vi "LSMcontroller_v66_improvedwfhandling.vi"() -> ()   [LabVIEW 2015] (continued)
                                in-place-border: w4031 -> [w4041]
                                in-place-border: [w4038] -> w4028
                                in-place-border: [w4037] -> w4027
                                n1319 = in-place-cluster #25(w4032) -> ("aDO"=w4040:u32[])
                                n1320 = call "remove channel from active arrayv2.vi"("line array in"=w4040, "line to remove"=w4041) -> ("line array out"=w4039:u32[], "removal"=w4038:bool, "index"=w4037:i32)
                                n1321 = in-place-cluster #25("aDO"=w4039) -> (w4029:T10)
                                }
                                n1322 = call "2pparameters.vi"("Params in"=w4029, "command"="set") -> ()  [unwired: 1 out]
                                }
                                frame True {
                                }
                                }
                                }
                                frame True {
                                n1323 = call "configuration.vi"("command"="get") -> ("config out"=w4048:T11)  [unwired: 2 in, 1 out]
                                n1324 = call "2pparameters.vi"("command"="get") -> ("params out"=w4052:T10)  [unwired: 1 in]
                                n1325 = Unbundle By Name(w4048) -> ("2P shutter"=w4047:i32)
                                n1326 = in-place {
                                in-place-border: w4047 -> [w4058]
                                in-place-border: [w4055] -> w4046
                                in-place-border: [w4054] -> w4044
                                n1327 = in-place-cluster #26(w4052) -> ("aDO"=w4057:u32[])
                                n1328 = call "add channel to active arrayv2.vi"("line array in"=w4057, "line to add"=w4058) -> ("line array out"=w4056:u32[], "addition"=w4055:bool, "index"=w4054:i32)
                                n1329 = in-place-cluster #26("aDO"=w4056) -> (w4050:T10)
                                }
                                n1330 = call "2pparameters.vi"("Params in"=w4050, "command"="set") -> ()  [unwired: 1 out]
                                }
                                }
                                }
                                frame #3 {
                                n1331 = local read "Measurement"() -> (w4062:T4)
                                n1332 = To Unsigned Long Integer(number=w4062) -> (unsigned 32bit integer=w4063:u32)
                                n1333 = case shown="5..7" w4063 {
                                tunnel: [FALSE ("addition") w4081] -> w4061
                                tunnel: [w4066 FALSE ("removal")] -> w4060
                                tunnel: [w4064 w4079] -> w4059
                                frame 0..4, Default {
                                n1334 = call "configuration.vi"("command"="get") -> ("config out"=w4072:T11)  [unwired: 2 in, 1 out]
                                n1335 = Unbundle By Name(w4072) -> ("LT timestamp"=w4069:u32)
                                n1336 = call "2pparameters.vi"("command"="get") -> ("params out"=w4070:T10)  [unwired: 1 in]
                                n1337 = in-place {
                                in-place-border: w4069 -> [w4078]
                                in-place-border: [w4075] -> w4066
                                in-place-border: [w4074] -> w4064
                                n1338 = in-place-cluster #27(w4070) -> ("aDO"=w4077:u32[])
                                n1339 = call "remove channel from active arrayv2.vi"("line array in"=w4077, "line to remove"=w4078) -> ("line array out"=w4076:u32[], "removal"=w4075:bool, "index"=w4074:i32)
                                n1340 = in-place-cluster #27("aDO"=w4076) -> (w4067:T10)
                                }
                                n1341 = call "2pparameters.vi"("Params in"=w4067, "command"="set") -> ()  [unwired: 1 out]
                                }
                                frame 5..7 {
                                n1342 = call "configuration.vi"("command"="get") -> ("config out"=w4087:T11)  [unwired: 2 in, 1 out]
                                n1343 = Unbundle By Name(w4087) -> ("LT timestamp"=w4084:u32)
                                n1344 = call "2pparameters.vi"("command"="get") -> ("params out"=w4085:T10)  [unwired: 1 in]
                                n1345 = in-place {
                                in-place-border: w4084 -> [w4093]
                                in-place-border: [w4090] -> w4081
                                in-place-border: [w4089] -> w4079
                                n1346 = in-place-cluster #28(w4085) -> ("aDO"=w4092:u32[])
                                n1347 = call "add channel to active arrayv2.vi"("line array in"=w4092, "line to add"=w4093) -> ("line array out"=w4091:u32[], "addition"=w4090:bool, "index"=w4089:i32)
                                n1348 = in-place-cluster #28("aDO"=w4091) -> (w4082:T10)
                                }
                                n1349 = call "2pparameters.vi"("Params in"=w4082, "command"="set") -> ()  [unwired: 1 out]
                                }
                                }
                                }
                                }
                                }
                                frame #1 {
                                n1350 = Or(x=w4100, y=w4101) -> (x .or. y?=w4099:bool)
                                n1351 = case shown="True" w4099 {
                                frame False {
                                }
                                frame True {
                                # "update GUI"
                                n1352 = call "Used AO lines.vi"() -> ("used AO names"=w4105:string[], "used AO lines"=w4107:tag[])  [unwired: 2 in]
                                n1353 = control-ref of="Analog Lines Plot"() -> (w4106:refnum<vi>)
                                n1354 = local write "Analog Used Lines"(w4107) -> ()
                                n1355 = local write "Analog Used Names"(w4105) -> ()
                                n1356 = call "prepAOWaveplot.vi"("WaveformGraph in"=w4106, "Analog Used Names"=w4105) -> ()  [unwired: 1 in]
                                }
                                }
                                n1357 = Compound Arithmetic op=OR(w4097, w4096, w4095, w4094) -> (w4098:bool)
                                n1358 = case shown="True" w4098 {
                                frame False {
                                }
                                frame True {
                                n1359 = control-ref of="Digital Lines Plot"() -> (w4102:refnum<vi>)
                                n1360 = call "Used DO lines.vi"() -> ("used DO names"=w4103:string[], "used DO lines"=w4104:tag[])  [unwired: 2 in]
                                n1361 = local write "Digital Used Lines"(w4104) -> ()
                                n1362 = local write "Digital Used Names"(w4103) -> ()
                                n1363 = call "prepDOWaveplot.vi"("DigitalGraph in"=w4102, "used DO names"=w4103) -> ()  [unwired: 1 in]
                                }
                                }
                                }
                                frame #2 {
                                n1364 = case shown="False" w4111 {
                                tunnel: [w4114 w4140] -> w4110
                                tunnel: [w4113 w4138] -> w4109
                                tunnel: [w4112 _] -> w4108
                                frame False {
                                n1365 = stacked-sequence {
                                seq-local: [w4116 _] -> [_ w4131]
                                tunnel: [w4116 _] -> w4114
                                tunnel: [w4119 _] -> w4113
                                tunnel: [w4115 _] -> w4112
                                frame #0 {
                                n1366 = call "configuration.vi"("command"="get") -> ("config out"=w4127:T11)  [unwired: 2 in, 1 out]
                                n1367 = call "waveformparamsv2.vi"("command"="get") -> ("Params out"=w4121:T14)  [unwired: 4 in, 2 out]
                                n1368 = Unbundle By Name(w4127) -> ("Voltage to Xgalvo"=w4128:i32)
                                n1369 = call "2pparameters.vi"("command"="get") -> ("params out"=w4124:T10)  [unwired: 1 in]
                                n1370 = Unbundle By Name(w4121) -> ("AO parameters"=w4120:T15)
                                n1371 = Unbundle By Name(w4124) -> ("aAO"=w4125:u32[])
                                n1372 = call "waveformsAObuffer.vi"("command"="get") -> ("AO wf out"=w4117:waveform(dbl)[])  [unwired: 1 in]
                                n1373 = Search 1D Array(1D array=w4125, element=w4128) -> (index of element=w4116:i32)  [unwired: 1 in]
                                n1374 = Index Array(array=w4117, index=w4116) -> (element=w4115:waveform(dbl))
                                n1375 = Index Array(array=w4120, index=w4116) -> (element=w4119:T16)
                                }
                                frame #1 {
                                w4132 = 0.0 ("Step size (V)")
                                n1376 = local read "Meastab"() -> (w4130:enum32{"X-Y Image", "Linescan", "Timetrace"})
                                n1377 = case shown="\"X-Y Image\", Default" w4130 {
                                tunnel: [w4134 w4135] -> w4129
                                frame "X-Y Image", Default {
                                n1378 = local read "Sampling rate"() -> (w4134:dbl)
                                }
                                frame "Timetrace" {
                                n1379 = local read "srateAODOtt"() -> (w4135:dbl)
                                }
                                }
                                n1380 = call "replace AO XYwfparam.vi"("Baseline (V)"=w4132, "Start amplitude (V)"=w4132, "Cycles"=w4132, "Repeats"=w4132, "index of AO wave"=w4131, "Step size (V)"=w4132, "DC (%)"=w4132, "Sampling frequency (Hz)"=w4129, "Period (ms)"=w4132, "Cycle length (s)"=w4132, "Pulses"=w4132, "padding value"=w4132, "Matlab wave name"=path "xwave") -> ()  [unwired: 3 in]
                                }
                                }
                                }
                                frame True {
                                w4139 = 0.0 ("Repeats")
                                n1381 = local read "Meastab"() -> (w4137:enum32{"X-Y Image", "Linescan", "Timetrace"})
                                n1382 = case shown="\"X-Y Image\", Default" w4137 {
                                tunnel: [w4156 w4157] -> w4136
                                frame "X-Y Image", Default {
                                n1383 = local read "Sampling rate"() -> (w4156:dbl)
                                }
                                frame "Timetrace" {
                                n1384 = local read "srateAODOtt"() -> (w4157:dbl)
                                }
                                }
                                n1385 = call "2pparameters.vi"("command"="get") -> ("params out"=w4142:T10)  [unwired: 1 in]
                                n1386 = call "configuration.vi"("command"="get") -> ("config out"=w4145:T11)  [unwired: 2 in, 1 out]
                                n1387 = call "waveformparamsv2.vi"("command"="get") -> ("Params out"=w4153:T14)  [unwired: 4 in, 2 out]
                                n1388 = Unbundle By Name(w4145) -> ("Voltage to Xgalvo"=w4146:i32)
                                n1389 = Unbundle By Name(w4153) -> ("AO parameters"=w4150:T15)
                                n1390 = Unbundle By Name(w4142) -> ("aAO"=w4143:u32[])
                                n1391 = Search 1D Array(1D array=w4143, element=w4146) -> (index of element=w4140:i32)  [unwired: 1 in]
                                n1392 = Index Array(array=w4150, index=0) -> (element=w4151:T16)
                                n1393 = Bundle By Name(cluster=w4151, "AOtab"=-1.0 ("Repeats"), "Repeats"=w4139, "Cycles"=w4139, "Start amplitude (V)"=w4139, "Baseline (V)"=w4139, "Step size (V)"=w4139, "DC (%)"=w4139, "Sampling frequency (Hz)"=w4136, "Period (ms)"=w4139, "Offset (V)"=w4139, "Amplitude (V)"=w4139, "Frequency"=w4139, "Tri Repeats"=w4139, "phase shift (ms)"=w4139, "Pulses"=w4139, "Matlab wave file"=path "xwave", "padding value"=w4139) -> (w4138:T16)
                                n1394 = Build Array(w4138) -> (w4148:T15)
                                n1395 = call "waveformparamsv2.vi"("command"="add AO", "add AO"=w4148) -> ()  [unwired: 3 in, 3 out]
                                }
                                }
                                }
                                frame #3 {
                                n1396 = case shown="False" w4161 {
                                tunnel: [w4164 w4190] -> w4160
                                tunnel: [w4163 w4188] -> w4159
                                tunnel: [w4162 _] -> w4158
                                frame False {
                                n1397 = stacked-sequence {
                                seq-local: [w4166 _] -> [_ w4181]
                                tunnel: [w4166 _] -> w4164
                                tunnel: [w4169 _] -> w4163
                                tunnel: [w4165 _] -> w4162
                                frame #0 {
                                n1398 = call "configuration.vi"("command"="get") -> ("config out"=w4177:T11)  [unwired: 2 in, 1 out]
                                n1399 = call "waveformparamsv2.vi"("command"="get") -> ("Params out"=w4171:T14)  [unwired: 4 in, 2 out]
                                n1400 = Unbundle By Name(w4177) -> ("Voltage to Ygalvo"=w4178:i32)
                                n1401 = call "2pparameters.vi"("command"="get") -> ("params out"=w4174:T10)  [unwired: 1 in]
                                n1402 = Unbundle By Name(w4171) -> ("AO parameters"=w4170:T15)
                                n1403 = Unbundle By Name(w4174) -> ("aAO"=w4175:u32[])
                                n1404 = call "waveformsAObuffer.vi"("command"="get") -> ("AO wf out"=w4167:waveform(dbl)[])  [unwired: 1 in]
                                n1405 = Search 1D Array(1D array=w4175, element=w4178) -> (index of element=w4166:i32)  [unwired: 1 in]
                                n1406 = Index Array(array=w4167, index=w4166) -> (element=w4165:waveform(dbl))
                                n1407 = Index Array(array=w4170, index=w4166) -> (element=w4169:T16)
                                }
                                frame #1 {
                                w4182 = 0.0 ("Step size (V)")
                                n1408 = local read "Meastab"() -> (w4180:enum32{"X-Y Image", "Linescan", "Timetrace"})
                                n1409 = case shown="\"X-Y Image\", Default" w4180 {
                                tunnel: [w4184 w4185] -> w4179
                                frame "X-Y Image", Default {
                                n1410 = local read "Sampling rate"() -> (w4184:dbl)
                                }
                                frame "Timetrace" {
                                n1411 = local read "srateAODOtt"() -> (w4185:dbl)
                                }
                                }
                                n1412 = call "replace AO XYwfparam.vi"("Baseline (V)"=w4182, "Start amplitude (V)"=w4182, "Cycles"=w4182, "Repeats"=w4182, "index of AO wave"=w4181, "Step size (V)"=w4182, "DC (%)"=w4182, "Sampling frequency (Hz)"=w4179, "Period (ms)"=w4182, "Cycle length (s)"=w4182, "Pulses"=w4182, "padding value"=w4182, "Matlab wave name"=path "ywave") -> ()  [unwired: 3 in]
                                }
                                }
                                }
                                frame True {
                                w4189 = 0.0 ("Repeats")
                                n1413 = local read "Meastab"() -> (w4187:enum32{"X-Y Image", "Linescan", "Timetrace"})
                                n1414 = case shown="\"X-Y Image\", Default" w4187 {
                                tunnel: [w4206 w4207] -> w4186
                                frame "X-Y Image", Default {
                                n1415 = local read "Sampling rate"() -> (w4206:dbl)
                                }
                                frame "Timetrace" {
                                n1416 = local read "srateAODOtt"() -> (w4207:dbl)
                                }
                                }
                                n1417 = call "2pparameters.vi"("command"="get") -> ("params out"=w4192:T10)  [unwired: 1 in]
                                n1418 = call "configuration.vi"("command"="get") -> ("config out"=w4195:T11)  [unwired: 2 in, 1 out]
                                n1419 = call "waveformparamsv2.vi"("command"="get") -> ("Params out"=w4204:T14)  [unwired: 4 in, 2 out]
                                n1420 = Unbundle By Name(w4195) -> ("Voltage to Ygalvo"=w4196:i32)
                                n1421 = Unbundle By Name(w4204) -> ("AO parameters"=w4201:T15)
                                n1422 = Unbundle By Name(w4192) -> ("aAO"=w4193:u32[])
                                n1423 = Search 1D Array(1D array=w4193, element=w4196) -> (index of element=w4190:i32)  [unwired: 1 in]
                                n1424 = Index Array(array=w4201, index=0) -> (element=w4202:T16)
                                n1425 = Bundle By Name(cluster=w4202, "AOtab"=-1.0 ("Repeats"), "Repeats"=w4189, "Cycles"=w4189, "Start amplitude (V)"=w4189, "Baseline (V)"=w4189, "Step size (V)"=w4189, "DC (%)"=w4189, "Sampling frequency (Hz)"=w4186, "Period (ms)"=w4189, "Offset (V)"=w4189, "Amplitude (V)"=w4189, "Frequency"=w4189, "Tri Repeats"=w4189, "phase shift (ms)"=w4189, "Pulses"=w4189, "Matlab wave file"=path "ywave", "padding value"=w4189) -> (w4188:T16)
                                n1426 = Build Array(w4188) -> (w4199:T15)
                                n1427 = call "waveformparamsv2.vi"("command"="add AO", "add AO"=w4199) -> ()  [unwired: 3 in, 3 out]
                                }
                                }
                                }
                                frame #4 {
                                n1428 = call "2pparameters.vi"("command"="get") -> ("params out"=w4213:T10)  [unwired: 1 in]
                                n1429 = Unbundle By Name(w4213) -> ("wavdet"=w4212:bool, "Pel"=w4209:sgl, "refwfsize"=w4208:dbl, "srateAODO"=w4211:sgl)
                                n1430 = case shown="True" w4212 {
                                tunnel: [w4217 w4227] -> w4215
                                tunnel: w4211 -> [w4218 w4229]
                                tunnel: w4209 -> [_ w4225]
                                tunnel: w4208 -> [_ w4224]
                                frame False {
                                n1431 = call "X-array-databuffer.vi"("command"=enum16{"get", "set", "clear", "append"}."get") -> ("array out"=w4221:dbl[])  [unwired: 3 in, 1 out]
                                n1432 = Reciprocal(x=w4218) -> (1/x=w4219:sgl)
                                n1433 = Bundle By Name("Y"=w4221, "dt"=w4219) -> (w4217:waveform(dbl))  [unwired: 1 in]
                                }
                                frame True {
                                n1434 = To Double Precision Float(number=w4225) -> (double precision float=w4226:dbl)
                                n1435 = Divide(x=w4224, y=w4226) -> (x/y=w4223:dbl)
                                n1436 = Round Toward +Infinity(x=w4223) -> (ceil(x): smallest int >= x=w4222:dbl)
                                n1437 = call "X-array-databuffer.vi"("command"=enum16{"get", "set", "clear", "append"}."get") -> ("array out"=w4231:dbl[])  [unwired: 3 in, 1 out]
                                n1438 = Reciprocal(x=w4229) -> (1/x=w4230:sgl)
                                n1439 = for {
                                N: w4222 -> [_]
                                tunnel: w4231 -> [w4233]
                                tunnel: [w4233] -> w4228 mode=concatenating
                                }
                                n1440 = Bundle By Name("Y"=w4228, "dt"=w4230) -> (w4227:waveform(dbl))  [unwired: 1 in]
                                }
                                }
                                n1441 = case shown="True" w4216 {
                                tunnel: w4215 -> [w4235 w4241]
                                tunnel: w4210 -> [w4236 _]
                                frame False {
                                n1442 = call "waveformsAObuffer.vi"("command"="get") -> ("AO wf out"=w4239:waveform(dbl)[])  [unwired: 1 in]
                                n1443 = property on="refwf" class="Ring (strict)" props=["RingText", "Text"]() -> ()  [unwired: 2 in, 3 out]
                                n1444 = Replace Array Subset(array=w4239, new element=w4235, index=w4236) -> (w4234:waveform(dbl)[])
                                n1445 = call "waveformsAObuffer.vi"("AO wf in"=w4234, "command"="set") -> ()  [unwired: 1 out]
                                }
                                frame True {
                                n1446 = call "waveformsAObuffer.vi"("command"="get") -> ("AO wf out"=w4243:waveform(dbl)[])  [unwired: 1 in]
                                n1447 = Build Array (concatenate)(w4243, w4241) -> (w4240:waveform(dbl)[])
                                n1448 = call "waveformsAObuffer.vi"("AO wf in"=w4240, "command"="set") -> ()  [unwired: 1 out]
                                }
                                }
                                }
                                frame #5 {
                                n1449 = call "2pparameters.vi"("command"="get") -> ("params out"=w4255:T10)  [unwired: 1 in]
                                n1450 = Unbundle By Name(w4255) -> ("wavdet"=w4254:bool, "Pel"=w4252:sgl, "refwfsize"=w4253:dbl, "srateAODO"=w4248:sgl)
                                n1451 = To Double Precision Float(number=w4252) -> (double precision float=w4251:dbl)
                                n1452 = Divide(x=w4253, y=w4251) -> (x/y=w4250:dbl)
                                n1453 = Round Toward +Infinity(x=w4250) -> (ceil(x): smallest int >= x=w4249:dbl)
                                n1454 = case shown="True" w4254 {
                                tunnel: [w4259 w4265] -> w4245
                                tunnel: w4249 -> [_ w4262]
                                tunnel: w4248 -> [w4260 w4267]
                                frame False {
                                n1455 = call "Y-array-databuffer.vi"("command"=enum16{"get", "set", "clear", "append"}."get") -> ("array out"=w4257:dbl[])  [unwired: 3 in, 1 out]
                                n1456 = Reciprocal(x=w4260) -> (1/x=w4261:sgl)
                                n1457 = Bundle By Name("Y"=w4257, "dt"=w4261) -> (w4259:waveform(dbl))  [unwired: 1 in]
                                }
                                frame True {
                                n1458 = call "Y-array-databuffer.vi"("command"=enum16{"get", "set", "clear", "append"}."get") -> ("array out"=w4263:dbl[])  [unwired: 3 in, 1 out]
                                n1459 = Reciprocal(x=w4267) -> (1/x=w4268:sgl)
                                n1460 = for {
                                N: w4262 -> [_]
                                tunnel: w4263 -> [w4269]
                                tunnel: [w4269] -> w4266 mode=concatenating
                                }
                                n1461 = Bundle By Name("Y"=w4266, "dt"=w4268) -> (w4265:waveform(dbl))  [unwired: 1 in]
                                }
                                }
                                n1462 = case shown="False" w4247 {
                                tunnel: w4245 -> [w4272 w4277]
                                tunnel: w4246 -> [w4273 _]
                                frame False {
                                n1463 = call "waveformsAObuffer.vi"("command"="get") -> ("AO wf out"=w4275:waveform(dbl)[])  [unwired: 1 in]
                                n1464 = Replace Array Subset(array=w4275, new element=w4272, index=w4273) -> (w4270:waveform(dbl)[])
                                n1465 = call "waveformsAObuffer.vi"("AO wf in"=w4270, "command"="set") -> ()  [unwired: 1 out]
                                }
                                frame True {
                                n1466 = call "waveformsAObuffer.vi"("command"="get") -> ("AO wf out"=w4279:waveform(dbl)[])  [unwired: 1 in]
                                n1467 = Build Array (concatenate)(w4279, w4277) -> (w4276:waveform(dbl)[])
                                n1468 = call "waveformsAObuffer.vi"("AO wf in"=w4276, "command"="set") -> ()  [unwired: 1 out]
                                }
                                }
                                }
                                frame #6 {
                                n1469 = Build Array(w4284, w4283) -> (w4287:bool[])
                                n1470 = Boolean Array To Number(Boolean array=w4287) -> (number=w4286:u32)
                                n1471 = case shown="2" w4286 {
                                tunnel: w4285 -> [_ _ _ _]
                                tunnel: w4282 -> [_ w4310 _ w4323]
                                tunnel: [_ w4309 _ w4320] -> w4281
                                frame 1 {
                                w4297 = 0.0 ("DOtab")
                                n1472 = call "2pparameters.vi"("command"="get") -> ("params out"=w4294:T10)  [unwired: 1 in]
                                n1473 = call "waveformparamsv2.vi"("command"="get") -> ("Params out"=w4305:T14)  [unwired: 4 in, 2 out]
                                n1474 = Unbundle By Name(w4305) -> ("DO parameters"=w4303:T17)
                                n1475 = Unbundle By Name(w4294) -> ("srate"=w4290:sgl, "Pel"=w4293:sgl)
                                n1476 = To Double Precision Float(number=w4290) -> (double precision float=w4288:dbl)
                                n1477 = To Double Precision Float(number=w4290) -> (double precision float=w4289:dbl)
                                n1478 = To Double Precision Float(number=w4293) -> (double precision float=w4292:dbl)
                                n1479 = Divide(x=w4289, y=w4292) -> (x/y=w4291:dbl)
                                n1480 = Index Array(array=w4303, index=0) -> (element=w4302:T18)
                                n1481 = Bundle By Name(cluster=w4302, "Digital DC (%)"=100.0, "Digital phase"=w4297, "Digital Freq (Hz)"=w4291, "Sampling frequency (Hz)"=w4288, "Digital time offset (s)"=w4297, "padding value"=0.0, "matlab wave file"=path "2Pshutter", "DOtab"=0.0) -> (w4300:T18)
                                n1482 = Build Array(w4300) -> (w4299:T17)
                                n1483 = call "waveformparamsv2.vi"("command"="add DO", "add DO"=w4299) -> ()  [unwired: 3 in, 3 out]
                                }
                                frame 2 {
                                n1484 = call "waveformparamsv2.vi"("command"="get") -> ("Params out"=w4312:T14)  [unwired: 4 in, 2 out]
                                n1485 = in-place {
                                in-place-border: w4310 -> [w4316]
                                in-place-border: [w4315] -> w4309
                                n1486 = in-place-cluster #29(w4312) -> ("DO parameters"=w4318:T17)
                                n1487 = Delete From Array(array=w4318, length=1, index=w4316) -> (deleted portion=w4315:T17, array with subset deleted=w4317:T17)
                                n1488 = in-place-cluster #29("DO parameters"=w4317) -> (w4311:T14)
                                }
                                n1489 = call "waveformparamsv2.vi"("command"="set", "Params in"=w4311) -> ()  [unwired: 3 in, 3 out]
                                }
                                frame 3, Default {
                                }
                                frame 0 {
                                n1490 = call "2pparameters.vi"("command"="get") -> ("params out"=w4325:T10)  [unwired: 1 in]
                                n1491 = Unbundle By Name(w4325) -> ("wavdet"=w4322:bool, "autoshutter"=w4324:bool)
                                n1492 = case shown="True" w4324 {
                                tunnel: w4323 -> [_ w4329]
                                tunnel: w4322 -> [_ w4328]
                                tunnel: [_ w4327] -> w4321
                                frame False {
                                }
                                frame True {
                                n1493 = case shown="False" w4328 {
                                tunnel: w4329 -> [w4331 _]
                                tunnel: [w4330 _] -> w4327
                                frame False {
                                n1494 = stacked-sequence {
                                tunnel: w4331 -> [w4333 w4347]
                                tunnel: [w4332 _] -> w4330
                                frame #0 {
                                n1495 = call "waveformparamsv2.vi"("command"="get") -> ("Params out"=w4335:T14)  [unwired: 4 in, 2 out]
                                n1496 = Unbundle By Name(w4335) -> ("DO parameters"=w4334:T17)
                                n1497 = Index Array(array=w4334, index=w4333) -> (element=w4332:T18)
                                }
                                frame #1 {
                                w4346 = 0.0 ("padding value")
                                n1498 = call "2pparameters.vi"("command"="get") -> ("params out"=w4344:T10)  [unwired: 1 in]
                                n1499 = Unbundle By Name(w4344) -> ("srate"=w4341:sgl, "Pel"=w4343:sgl)
                                n1500 = To Double Precision Float(number=w4341) -> (double precision float=w4339:dbl)
                                n1501 = To Double Precision Float(number=w4341) -> (double precision float=w4340:dbl)
                                n1502 = To Double Precision Float(number=w4343) -> (double precision float=w4342:dbl)
                                n1503 = Divide(x=w4340, y=w4342) -> (x/y=w4338:dbl)
                                n1504 = call "replace DO wf param.vi"("Digital Freq (Hz)"=w4338, "Digital DC (%)"=100.0, "Digital phase"=w4346, "Sampling frequency (Hz)"=w4339, "Digital time offset (s)"=w4346, "index of DO wave"=w4347, "padding value"=w4346, "matlab wave file"=path "2Pshutter" ("matlab wave number")) -> ()  [unwired: 3 in]
                                }
                                }
                                }
                                frame True {
                                }
                                }
                                }
                                }
                                n1505 = Build Array(w4321) -> (w4320:T17)
                                }
                                }
                                }
                                frame #7 {
                                n1506 = Build Array(w4352, w4351) -> (w4354:bool[])
                                n1507 = Boolean Array To Number(Boolean array=w4354) -> (number=w4353:u32)
                                n1508 = case shown="0" w4353 {
                                tunnel: w4350 -> [_ w4396 _ w4403]
                                tunnel: [_ w4395 _ w4401] -> w4349
                                frame 1 {
                                n1509 = call "2pparameters.vi"("command"="get") -> ("params out"=w4361:T10)  [unwired: 1 in]
                                n1510 = Unbundle By Name(w4361) -> ("wavdet"=w4362:bool, "Pel"=w4364:sgl, "refwfsize"=w4365:dbl, "srateAODO"=w4363:sgl)
                                n1511 = call "waveformsDObuffer.vi"("command"="get") -> ("DO wf out"=w4357:digitalwaveform[])  [unwired: 1 in]
                                n1512 = case shown="False" w4362 {
                                tunnel: [w4370 w4380] -> w4359
                                tunnel: w4363 -> [w4375 w4391]
                                tunnel: w4364 -> [w4369 w4384]
                                tunnel: w4365 -> [_ w4388]
                                frame False {
                                w4373 = u16 0 items=["unsigned binary", "offset binary", "2's complement"] ("data format (offset binary)")
                                n1513 = Initialize Array(sgl 1.0, w4369) -> (w4366:sgl[])
                                n1514 = Reciprocal(x=w4375) -> (1/x=w4376:sgl)
                                n1515 = Bundle By Name("Y"=w4366, "dt"=w4376) -> (w4371:waveform(sgl))  [unwired: 1 in]
                                n1516 = call-poly <vilib>:"Analog to Digital.vi"("data format (offset binary)"=w4373, "compress digital (T)"=TRUE, "full-scale range (pk-pk)"=1.0, "resolution (16 bit)"=1, "analog waveform"=w4371) -> ("digital waveform"=w4370:digitalwaveform)  [unwired: 3 in, 3 out]
                                }
                                frame True {
                                w4383 = u16 0 items=["unsigned binary", "offset binary", "2's complement"] ("data format (offset binary)")
                                n1517 = To Double Precision Float(number=w4384) -> (double precision float=w4389:dbl)
                                n1518 = Initialize Array(sgl 1.0, w4384) -> (w4377:sgl[])
                                n1519 = Divide(x=w4388, y=w4389) -> (x/y=w4386:dbl)
                                n1520 = Round Toward +Infinity(x=w4386) -> (ceil(x): smallest int >= x=w4387:dbl)
                                n1521 = for {
                                N: w4387 -> [_]
                                tunnel: w4377 -> [w4393]
                                tunnel: [w4393] -> w4390 mode=concatenating
                                }
                                n1522 = Reciprocal(x=w4391) -> (1/x=w4392:sgl)
                                n1523 = Bundle By Name("Y"=w4390, "dt"=w4392) -> (w4381:waveform(sgl))  [unwired: 1 in]
                                n1524 = call-poly <vilib>:"Analog to Digital.vi"("data format (offset binary)"=w4383, "compress digital (T)"=TRUE, "full-scale range (pk-pk)"=1.0, "resolution (16 bit)"=1, "analog waveform"=w4381) -> ("digital waveform"=w4380:digitalwaveform)  [unwired: 3 in, 3 out]
                                }
                                }
                                n1525 = Build Array (concatenate)(w4357, w4359) -> (w4355:digitalwaveform[])
                                n1526 = call "waveformsDObuffer.vi"("DO wf in"=w4355, "command"="set") -> ()  [unwired: 1 out]
                                }
                                frame 2 {
                                n1527 = call "waveformsDObuffer.vi"("command"="get") -> ("DO wf out"=w4398:digitalwaveform[])  [unwired: 1 in]
                                n1528 = Delete From Array(array=w4398, length=1, index=w4396) -> (deleted portion=w4395:digitalwaveform[], array with subset deleted=w4394:digitalwaveform[])
                                n1529 = call "waveformsDObuffer.vi"("DO wf in"=w4394, "command"="set") -> ()  [unwired: 1 out]
                                }
                                frame 3, Default {
                                }
                                frame 0 {
                                n1530 = call "2pparameters.vi"("command"="get") -> ("params out"=w4405:T10)  [unwired: 1 in]
                                n1531 = Unbundle By Name(w4405) -> ("autoshutter"=w4404:bool, "wavdet"=w4402:bool)
                                n1532 = case shown="True" w4404 {
                                tunnel: w4403 -> [_ w4409]
                                tunnel: w4402 -> [_ w4408]
                                tunnel: [_ w4407] -> w4401
                                frame False {
                                }
                                frame True {
                                n1533 = case shown="False" w4408 {
                                tunnel: w4409 -> [w4413 _]
                                tunnel: [w4411 _] -> w4407
                                frame False {
                                w4420 = u16 0 items=["unsigned binary", "offset binary", "2's complement"] ("data format (offset binary)")
                                n1534 = call "2pparameters.vi"("command"="get") -> ("params out"=w4427:T10)  [unwired: 1 in]
                                n1535 = call "waveformsDObuffer.vi"("command"="get") -> ("DO wf out"=w4414:digitalwaveform[])  [unwired: 1 in]
                                n1536 = Unbundle By Name(w4427) -> ("Pel"=w4429:sgl, "srate"=w4428:sgl)
                                n1537 = Index Array(array=w4414, index=w4413) -> (element=w4412:digitalwaveform)
                                n1538 = Build Array(w4412) -> (w4411:digitalwaveform[])
                                n1539 = Initialize Array(sgl 1.0, w4429) -> (w4415:sgl[])
                                n1540 = Reciprocal(x=w4428) -> (1/x=w4422:sgl)
                                n1541 = Bundle By Name("Y"=w4415, "dt"=w4422) -> (w4418:waveform(sgl))  [unwired: 1 in]
                                n1542 = call-poly <vilib>:"Analog to Digital.vi"("data format (offset binary)"=w4420, "compress digital (T)"=TRUE, "full-scale range (pk-pk)"=1.0, "resolution (16 bit)"=1, "analog waveform"=w4418) -> ("digital waveform"=w4425:digitalwaveform)  [unwired: 3 in, 3 out]
                                n1543 = Replace Array Subset(array=w4414, new element=w4425, index=w4413) -> (w4410:digitalwaveform[])
                                n1544 = call "waveformsDObuffer.vi"("DO wf in"=w4410, "command"="set") -> ()  [unwired: 1 out]
                                }
                                frame True {
                                }
                                }
                                }
                                }
                                }
                                }
                                }
                                frame #8 {
                                n1545 = Build Array(w4433, w4432) -> (w4435:bool[])
                                n1546 = Boolean Array To Number(Boolean array=w4435) -> (number=w4434:u32)
                                n1547 = case shown="0" w4434 {
                                tunnel: w4431 -> [_ w4461 _ w4473]
                                tunnel: [_ w4460 _ w4471] -> w4430
                                frame 1 {
                                w4448 = 0.0 ("DOtab")
                                n1548 = call "2pparameters.vi"("command"="get") -> ("params out"=w4446:T10)  [unwired: 1 in]
                                n1549 = call "waveformparamsv2.vi"("command"="get") -> ("Params out"=w4456:T14)  [unwired: 4 in, 2 out]
                                n1550 = Unbundle By Name(w4456) -> ("DO parameters"=w4454:T17)
                                n1551 = Unbundle By Name(w4446) -> ("srate"=w4443:sgl, "Pel"=w4445:sgl)
                                n1552 = To Double Precision Float(number=w4443) -> (double precision float=w4441:dbl)
                                n1553 = To Double Precision Float(number=w4443) -> (double precision float=w4442:dbl)
                                n1554 = To Double Precision Float(number=w4445) -> (double precision float=w4437:dbl)
                                n1555 = Divide(x=w4442, y=w4437) -> (x/y=w4444:dbl)
                                n1556 = Index Array(array=w4454, index=0) -> (element=w4453:T18)
                                n1557 = Divide(x=1.0 ("Digital DC (%)"), y=w4437) -> (x/y=w4439:dbl)
                                n1558 = Multiply(x=100.0, y=w4439) -> (x*y=w4436:dbl)
                                n1559 = Bundle By Name(cluster=w4453, "Digital DC (%)"=w4436, "Digital phase"=w4448, "Digital Freq (Hz)"=w4444, "Sampling frequency (Hz)"=w4441, "Digital time offset (s)"=w4448, "padding value"=0.0, "matlab wave file"=path "LT", "DOtab"=0.0) -> (w4451:T18)
                                n1560 = Build Array(w4451) -> (w4450:T17)
                                n1561 = call "waveformparamsv2.vi"("command"="add DO", "add DO"=w4450) -> ()  [unwired: 3 in, 3 out]
                                }
                                frame 2 {
                                n1562 = call "waveformparamsv2.vi"("command"="get") -> ("Params out"=w4463:T14)  [unwired: 4 in, 2 out]
                                n1563 = in-place {
                                in-place-border: w4461 -> [w4467]
                                in-place-border: [w4466] -> w4460
                                n1564 = in-place-cluster #30(w4463) -> ("DO parameters"=w4469:T17)
                                n1565 = Delete From Array(array=w4469, length=1, index=w4467) -> (deleted portion=w4466:T17, array with subset deleted=w4468:T17)
                                n1566 = in-place-cluster #30("DO parameters"=w4468) -> (w4462:T14)
                                }
                                n1567 = call "waveformparamsv2.vi"("command"="set", "Params in"=w4462) -> ()  [unwired: 3 in, 3 out]
                                }
                                frame 3, Default {
                                }
                                frame 0 {
                                n1568 = local read "Measurement"() -> (w4475:T4)
                                n1569 = To Unsigned Long Integer(number=w4475) -> (unsigned 32bit integer=w4474:u32)
                                n1570 = case shown="5..7" w4474 {
                                tunnel: w4473 -> [_ w4477]
                                tunnel: [_ w4476] -> w4472
                                frame 0..4, Default {
                                }
                                frame 5..7 {
                                n1571 = stacked-sequence {
                                tunnel: w4477 -> [w4479 w4488]
                                tunnel: [w4478 _] -> w4476
                                frame #0 {
                                n1572 = call "waveformparamsv2.vi"("command"="get") -> ("Params out"=w4481:T14)  [unwired: 4 in, 2 out]
                                n1573 = Unbundle By Name(w4481) -> ("DO parameters"=w4482:T17)
                                n1574 = Index Array(array=w4482, index=w4479) -> (element=w4478:T18)
                                }
                                frame #1 {
                                w4496 = 0.0 ("padding value")
                                n1575 = call "2pparameters.vi"("command"="get") -> ("params out"=w4494:T10)  [unwired: 1 in]
                                n1576 = Unbundle By Name(w4494) -> ("srate"=w4492:sgl, "Pel"=w4493:sgl)
                                n1577 = To Double Precision Float(number=w4492) -> (double precision float=w4490:dbl)
                                n1578 = To Double Precision Float(number=w4492) -> (double precision float=w4491:dbl)
                                n1579 = To Double Precision Float(number=w4493) -> (double precision float=w4486:dbl)
                                n1580 = Divide(x=1.0 ("Digital DC (%)"), y=w4486) -> (x/y=w4485:dbl)
                                n1581 = Multiply(x=100.0, y=w4485) -> (x*y=w4484:dbl)
                                n1582 = Divide(x=w4491, y=w4486) -> (x/y=w4489:dbl)
                                n1583 = call "replace DO wf param.vi"("Digital Freq (Hz)"=w4489, "Digital DC (%)"=w4484, "Digital phase"=w4496, "Sampling frequency (Hz)"=w4490, "Digital time offset (s)"=w4496, "index of DO wave"=w4488, "padding value"=w4496, "matlab wave file"=path "LT" ("matlab wave number")) -> ()  [unwired: 3 in]
                                }
                                }
                                }
                                }
                                n1584 = Build Array(w4472) -> (w4471:T17)
                                }
                                }
                                }
                                frame #9 {
                                n1585 = Build Array(w4501, w4500) -> (w4503:bool[])
                                n1586 = Boolean Array To Number(Boolean array=w4503) -> (number=w4502:u32)
                                n1587 = case shown="0" w4502 {
                                tunnel: w4499 -> [_ w4555 _ w4559]
                                tunnel: [_ w4550 _ w4556] -> w4498
                                frame 1 {
                                n1588 = call "2pparameters.vi"("command"="get") -> ("params out"=w4510:T10)  [unwired: 1 in]
                                n1589 = Unbundle By Name(w4510) -> ("wavdet"=w4511:bool, "Pel"=w4513:sgl, "refwfsize"=w4514:dbl, "Pel"=w4512:sgl)
                                n1590 = call "waveformsDObuffer.vi"("command"="get") -> ("DO wf out"=w4506:digitalwaveform[])  [unwired: 1 in]
                                n1591 = case shown="True" w4511 {
                                tunnel: [w4518 w4531] -> w4508
                                tunnel: w4512 -> [w4527 w4546]
                                tunnel: w4513 -> [w4517 w4537]
                                tunnel: w4514 -> [_ w4543]
                                frame False {
                                w4521 = u16 0 items=["unsigned binary", "offset binary", "2's complement"] ("data format (offset binary)")
                                n1592 = Initialize Array(sgl 0.0, w4517) -> (w4524:sgl[])
                                n1593 = Replace Array Subset(array=w4524, new element=sgl 1.0, index=0) -> (w4522:sgl[])
                                n1594 = Reciprocal(x=w4527) -> (1/x=w4528:sgl)
                                n1595 = Bundle By Name("Y"=w4522, "dt"=w4528) -> (w4519:waveform(sgl))  [unwired: 1 in]
                                n1596 = call-poly <vilib>:"Analog to Digital.vi"("data format (offset binary)"=w4521, "compress digital (T)"=TRUE, "full-scale range (pk-pk)"=1.0, "resolution (16 bit)"=1, "analog waveform"=w4519) -> ("digital waveform"=w4518:digitalwaveform)  [unwired: 3 in, 3 out]
                                }
                                frame True {
                                w4534 = u16 0 items=["unsigned binary", "offset binary", "2's complement"] ("data format (offset binary)")
                                n1597 = To Double Precision Float(number=w4537) -> (double precision float=w4544:dbl)
                                n1598 = Initialize Array(sgl 0.0, w4537) -> (w4539:sgl[])
                                n1599 = Divide(x=w4543, y=w4544) -> (x/y=w4541:dbl)
                                n1600 = Round Toward +Infinity(x=w4541) -> (ceil(x): smallest int >= x=w4542:dbl)
                                n1601 = Replace Array Subset(array=w4539, new element=sgl 1.0, index=0) -> (w4536:sgl[])
                                n1602 = for {
                                N: w4542 -> [_]
                                tunnel: w4536 -> [w4548]
                                tunnel: [w4548] -> w4545 mode=concatenating
                                }
                                n1603 = Reciprocal(x=w4546) -> (1/x=w4547:sgl)
                                n1604 = Bundle By Name("Y"=w4545, "dt"=w4547) -> (w4532:waveform(sgl))  [unwired: 1 in]
                                n1605 = call-poly <vilib>:"Analog to Digital.vi"("data format (offset binary)"=w4534, "compress digital (T)"=TRUE, "full-scale range (pk-pk)"=1.0, "resolution (16 bit)"=1, "analog waveform"=w4532) -> ("digital waveform"=w4531:digitalwaveform)  [unwired: 3 in, 3 out]
                                }
                                }
                                n1606 = Build Array (concatenate)(w4506, w4508) -> (w4504:digitalwaveform[])
                                n1607 = call "waveformsDObuffer.vi"("DO wf in"=w4504, "command"="set") -> ()  [unwired: 1 out]
                                }
                                frame 2 {
                                n1608 = call "waveformsDObuffer.vi"("command"="get") -> ("DO wf out"=w4552:digitalwaveform[])  [unwired: 1 in]
                                n1609 = Delete From Array(array=w4552, length=1, index=w4555) -> (deleted portion=w4550:digitalwaveform[], array with subset deleted=w4549:digitalwaveform[])
                                n1610 = call "waveformsDObuffer.vi"("DO wf in"=w4549, "command"="set") -> ()  [unwired: 1 out]
                                }
                                frame 3, Default {
                                }
                                frame 0 {
                                n1611 = local read "Measurement"() -> (w4558:T4)
                                n1612 = To Unsigned Long Integer(number=w4558) -> (unsigned 32bit integer=w4557:u32)
                                n1613 = case shown="5..7" w4557 {
                                tunnel: w4559 -> [_ w4562]
                                tunnel: [_ w4561] -> w4556
                                frame 0..4, Default {
                                }
                                frame 5..7 {
                                n1614 = call "2pparameters.vi"("command"="get") -> ("params out"=w4569:T10)  [unwired: 1 in]
                                n1615 = Unbundle By Name(w4569) -> ("wavdet"=w4570:bool, "Pel"=w4572:sgl, "refwfsize"=w4573:dbl, "srateAODO"=w4571:sgl)
                                n1616 = call "waveformsDObuffer.vi"("command"="get") -> ("DO wf out"=w4563:digitalwaveform[])  [unwired: 1 in]
                                n1617 = Index Array(array=w4563, index=w4562) -> (element=w4564:digitalwaveform)
                                n1618 = case shown="True" w4570 {
                                tunnel: [w4577 w4590] -> w4567
                                tunnel: w4571 -> [w4586 w4605]
                                tunnel: w4572 -> [w4576 w4596]
                                tunnel: w4573 -> [_ w4602]
                                frame False {
                                w4580 = u16 0 items=["unsigned binary", "offset binary", "2's complement"] ("data format (offset binary)")
                                n1619 = Initialize Array(sgl 0.0, w4576) -> (w4583:sgl[])
                                n1620 = Replace Array Subset(array=w4583, new element=sgl 1.0, index=0) -> (w4581:sgl[])
                                n1621 = Reciprocal(x=w4586) -> (1/x=w4587:sgl)
                                n1622 = Bundle By Name("Y"=w4581, "dt"=w4587) -> (w4578:waveform(sgl))  [unwired: 1 in]
                                n1623 = call-poly <vilib>:"Analog to Digital.vi"("data format (offset binary)"=w4580, "compress digital (T)"=TRUE, "full-scale range (pk-pk)"=1.0, "resolution (16 bit)"=1, "analog waveform"=w4578) -> ("digital waveform"=w4577:digitalwaveform)  [unwired: 3 in, 3 out]
                                }
                                frame True {
                                w4593 = u16 0 items=["unsigned binary", "offset binary", "2's complement"] ("data format (offset binary)")
                                n1624 = To Double Precision Float(number=w4596) -> (double precision float=w4603:dbl)
                                n1625 = Initialize Array(sgl 0.0, w4596) -> (w4598:sgl[])
                                n1626 = Divide(x=w4602, y=w4603) -> (x/y=w4600:dbl)
                                n1627 = Round Toward +Infinity(x=w4600) -> (ceil(x): smallest int >= x=w4601:dbl)
                                n1628 = Replace Array Subset(array=w4598, new element=sgl 1.0, index=0) -> (w4595:sgl[])
                                n1629 = for {
                                N: w4601 -> [_]
                                tunnel: w4595 -> [w4607]
                                tunnel: [w4607] -> w4604 mode=concatenating
                                }
                                n1630 = Reciprocal(x=w4605) -> (1/x=w4606:sgl)
                                n1631 = Bundle By Name("Y"=w4604, "dt"=w4606) -> (w4591:waveform(sgl))  [unwired: 1 in]
                                n1632 = call-poly <vilib>:"Analog to Digital.vi"("data format (offset binary)"=w4593, "compress digital (T)"=TRUE, "full-scale range (pk-pk)"=1.0, "resolution (16 bit)"=1, "analog waveform"=w4591) -> ("digital waveform"=w4590:digitalwaveform)  [unwired: 3 in, 3 out]
                                }
                                }
                                n1633 = Build Array(w4564) -> (w4561:digitalwaveform[])
                                n1634 = Replace Array Subset(array=w4563, new element=w4567, index=w4562) -> (w4560:digitalwaveform[])
                                n1635 = call "waveformsDObuffer.vi"("DO wf in"=w4560, "command"="set") -> ()  [unwired: 1 out]
                                }
                                }
                                }
                                }
                                }
                                frame #10 {
                                n1636 = local read "Meastab"() -> (w4621:enum32{"X-Y Image", "Linescan", "Timetrace"})
                                n1637 = property on="refwf" class="Ring (strict)"() -> ("RingText.Text"=w4618:string)  [unwired: 2 in, 2 out]
                                n1638 = case shown="\"Timetrace\"" w4621 {
                                tunnel: [w4623 w4624] -> w4622
                                frame "X-Y Image", Default {
                                n1639 = local read "Sampling rate"() -> (w4623:dbl)
                                }
                                frame "Timetrace" {
                                n1640 = local read "srateAODOtt"() -> (w4624:dbl)
                                }
                                }
                                n1641 = call "waveformsAObuffer.vi"("command"="get") -> ("AO wf out"=w4611:waveform(dbl)[])  [unwired: 1 in]
                                n1642 = local read "wavdet"() -> (w4619:bool)
                                n1643 = call "waveformsDObuffer.vi"("command"="get") -> ("DO wf out"=w4615:digitalwaveform[])  [unwired: 1 in]
                                n1644 = call "correctwaveformsizetemp.vi"("new sampling frequency (Hz)"=w4622, "start"=TRUE, "reference waveforms to"=w4618, "Analog waveforms in"=w4611, "stop"=FALSE, "Digital waveforms in"=w4615) -> ("analog wf out"=w4617:waveform(dbl)[], "Digital wf out"=w4610:digitalwaveform[], "measpoints"=w4620:i32)
                                n1645 = call "waveformsDObuffer.vi"("DO wf in"=w4610, "command"="set") -> ()  [unwired: 1 out]
                                n1646 = call "waveformsAObuffer.vi"("AO wf in"=w4617, "command"="set") -> ()  [unwired: 1 out]
                                n1647 = case shown="True" w4619 {
                                tunnel: w4620 -> [_ w4627]
                                tunnel: w4610 -> [_ w4625]
                                frame False {
                                }
                                frame True {
                                n1648 = local write "# of frames"(w4627) -> ()
                                n1649 = call "GetNumCamFramesv2.vi"("Digital Waveform Graph"=w4625) -> ("Numeric"=w4626:i32)  [unwired: 10 in]
                                n1650 = local write "Total Camera Frames"(w4626) -> ()
                                }
                                }
                                }
                                }
                              }
                              frame #7 {
                                # "Disabled for conversion to 64 bit"
                                n1651 = disable-structure shown="Disabled" {
                                frame Disabled {
                                n1652 = local read "Measurement"() -> (w4629:T4)
                                n1653 = case shown="\"Lifetime (scan)\"" w4629 {
                                frame "X-Y-t movie", Default {
                                }
                                frame "Lifetime (scan)" {
                                # "total acquisition time"
                                n1654 = call "2pparameters.vi"("command"="get") -> ("params out"=w4637:T10)  [unwired: 1 in]
                                n1655 = Unbundle By Name(w4637) -> ("measpoints"=w4631:i32, "srateAODO"=w4652:sgl)
                                n1656 = Divide(x=w4631, y=w4652) -> (x/y=w4630:sgl)
                                n1657 = local read "min phot"() -> (w4647:u32)
                                n1658 = local read "expected c/s"() -> (w4648:dbl)
                                n1659 = Multiply(x=w4630, y=1000.0) -> (x*y=w4640:dbl)
                                n1660 = local read "Ch1 ZeroX"() -> (w4645:i32)
                                n1661 = local read "truncate"() -> (w4646:u32)
                                n1662 = To Long Integer(number=w4640) -> (32bit integer=w4649:i32)
                                n1663 = To Long Integer(number=w4648) -> (32bit integer=w4650:i32)
                                n1664 = local read "Number of Bins"() -> (w4641:u32)
                                n1665 = local read "Ch1 Level"() -> (w4643:i32)
                                n1666 = local read "Ch0 ZeroX"() -> (w4644:i32)
                                n1667 = local write "Acquisition time"(w4649) -> ()
                                n1668 = local read "Ch0 Level"() -> (w4642:i32)
                                n1669 = call "lifetimeparameters.vi"("command"="get") -> ("Params out"=w4635:T19)  [unwired: 1 in]
                                n1670 = Add(x=100, y=w4649) -> (x+y=w4639:i32)
                                n1671 = Bundle By Name(cluster=w4635, "acq time"=w4639, "acq rate"=w4650, "# bins"=w4641, "Ch0 Level"=w4642, "Ch1 Level"=w4643, "Ch0 ZeroX"=w4644, "Ch1 ZeroX"=w4645, "min photons"=w4647, "truncate"=w4646) -> (w4634:T19)
                                n1672 = local write "Acquisition rate"(w4650) -> ()
                                n1673 = call "lifetimeparameters.vi"("Params in"=w4634, "command"="set") -> ()  [unwired: 1 out]
                                }
                                }
                                }
                                frame Enabled {
                                }
                                }
                                n1674 = local write "64bit disabled"(TRUE ("64bit disabled")) -> ()
                              }
                              frame #8 {
                                n1675 = call "2pparameters.vi"("command"="get") -> ("params out"=w4663:T10)  [unwired: 1 in]
                                n1676 = Unbundle By Name(w4663) -> ("refreshbuffer"=w4661:i32, "srate"=w4662:sgl)
                                n1677 = local read "wavdet"() -> (w4653:bool)
                                n1678 = To Double Precision Float(number=w4662) -> (double precision float=w4665:dbl)
                                n1679 = To Double Precision Float(number=w4661) -> (double precision float=w4656:dbl)
                                n1680 = case shown="False" w4653 {
                                tunnel: [w4670 w4671] -> w4655
                                frame False {
                                w4670 = 10123 items=["Finite Samples"=10178, "Continuous Samples"=10123, "Hardware Timed Single Point"=12522] ("sample mode")
                                }
                                frame True {
                                w4671 = 10123 items=["Finite Samples"=10178, "Continuous Samples"=10123, "Hardware Timed Single Point"=12522] ("sample mode")
                                }
                                }
                                n1681 = Divide(x=w4656, y=w4665) -> (x/y=w4669:dbl)
                                n1682 = Multiply(x=w4669, y=2.0) -> (x*y=w4666:dbl)
                                n1683 = Max & Min(x=w4666, y=10.0) -> (max(x,y)=w4657:dbl)  [unwired: 1 out]
                                n1684 = call "2pparameters.vi"("command"="get") -> ("params out"=w4660:T10)  [unwired: 1 in]
                                n1685 = Bundle By Name(cluster=w4660, "timeout"=w4657, "sample mode"=w4655) -> (w4658:T10)
                                n1686 = call "2pparameters.vi"("Params in"=w4658, "command"="set") -> ()  [unwired: 1 out]
                              }
                            }
                          }
                          frame #1 {
                            # "Disabled for conversion to 64 bit"
                            n1687 = call "prepAO_img.vi"() -> ("Terminal Name with Device Prefix"=w4673:tag)
                            n1688 = call "prepDO_img.vi"() -> ()  [unwired: 2 in]
                            n1689 = call "prepAI_img.vi"("triggersource"=w4673) -> ()  [unwired: 2 in]
                            n1690 = call "prepCI_img.vi"("ArmStart.DigEdge.Src"=w4673) -> ()  [unwired: 1 in]
                            n1691 = disable-structure shown="Disabled" {
                              frame Disabled {
                                n1692 = local read "Measurement"() -> (w4674:T4)
                                n1693 = case shown="\"Lifetime (contour)\"" w4674 {
                                frame "X-Y-t movie", Default {
                                }
                                frame "Lifetime (contour)" {
                                n1694 = stacked-sequence {
                                frame #0 {
                                n1695 = call "PH-temp.vi"("String"="clear" ("command")) -> ()  [unwired: 2 in, 2 out]
                                n1696 = call "PH-temp-raw.vi"("command"="empty") -> ()  [unwired: 1 in, 1 out]
                                }
                                frame #1 {
                                n1697 = call "calib.vi"() -> ()  [unwired: 1 in]
                                }
                                frame #2 {
                                n1698 = call "setup.vi"() -> ()  [unwired: 1 in]
                                }
                                }
                                }
                                }
                              }
                              frame Enabled {
                              }
                            }
                            n1699 = local write "64bit disabled"(TRUE ("64bit disabled")) -> ()
                          }
                          frame #2 {
                            n1700 = local read "save\ndata"() -> (w4677:bool)
                            n1701 = case shown="True" w4677 {
                              tunnel: w4678 -> [_ w4682]
                              frame False {
                              }
                              frame True {
                                n1702 = local read "filename prefix"() -> (w4680:string)
                                n1703 = local read "data dir"() -> (w4681:path)
                                n1704 = call "preparebinaryfiles.vi"("filename prefix"=w4680, "data dir"=w4681, "timestamp"=w4682) -> ("full-filename"=w4679:string)  [unwired: 1 in]
                                n1705 = local write "full-filename"(w4679) -> ()
                              }
                            }
                            n1706 = call "preptempbuffers_tt.vi"() -> ()  [unwired: 12 in]
                          }
                          frame #3 {
                            n1707 = local read "wavdet"() -> (w4683:bool)
